vi "Simulation Lab While Loop B220061.vi"() -> ()   [LabVIEW 2020]
panel:
  in  "stop":bool
  out "Numeric 3":i32
  out "Numeric 2":dbl
  out "Numeric":dbl
  out "Tank":dbl(slide) scale=0.0..10.0
  in  "Slide 2":dbl(slide) scale=0.0..10.0
  in  "Slide":dbl(slide) scale=0.0..10.0
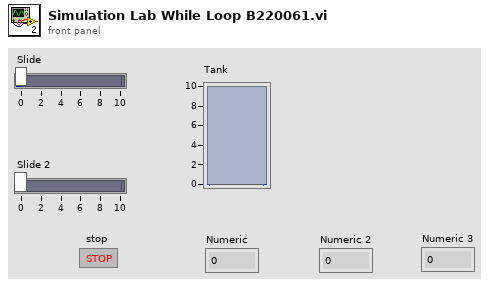
[diagram p1: front panel]
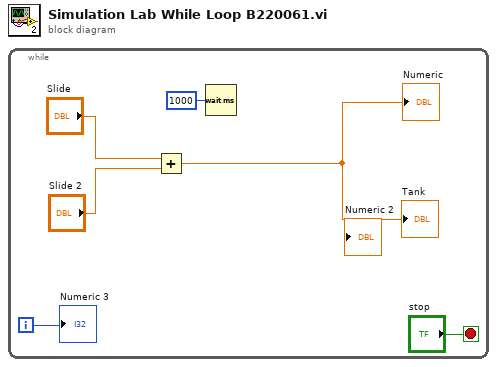
[diagram p0: block diagram]
diagram:
  n1 = while {
    i -> [w2]
    stop <- "stop" stop-if-true
    n2 = Add(x="Slide", y="Slide 2") -> (x+y=→"Tank" →"Numeric":dbl)
    n3 = Wait (ms)(milliseconds to wait=u32 1000) -> ()  [unwired: 1 out]
    "Numeric 3" <- w2
  }
